vi "PR_Update_screw_eve_result.vi"(8 "result":string, 9 "data":T1, 10 "barcode":string="984132195", 11 "DBlink":string="Driver={ODBC Driver 17 for SQL Server};Server=localhost\\SQLEXPRESS;Database=ZDX201;UID=labview;PWD=Dsa@54137926") -> (0 "error out":errorcluster)   [LabVIEW 2019]
uses:
  <vilib>/addons/database/Connection.llb/DB Tools Open Connec (String).vi
  <vilib>/addons/database/NI_Database_API.lvlib
panel:
  out "concatenated string":string="WHERE [barcode]='984132195' and [pos]='B'"
  in  "error in (no error)":errorcluster
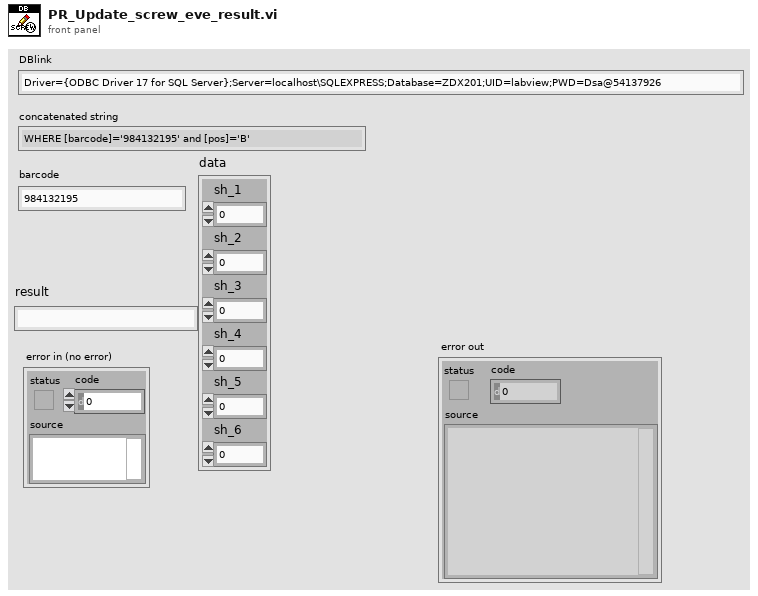
[diagram p1: front panel]
types:
  T1 = cluster{"sh_1":dbl, "sh_2":dbl, "sh_3":dbl, "sh_4":dbl, "sh_5":dbl, "sh_6":dbl}
  T2 = cluster{"done_time3":timestamp, "update_time":timestamp, "result":string, "sh_1":dbl, "sh_2":dbl, "sh_3":dbl, "sh_4":dbl, "sh_5":dbl, "sh_6":dbl}
  T3 = typedef "NI_Database_API.lvlib/Conn ObjectReference.ctl" = refnum<k1>
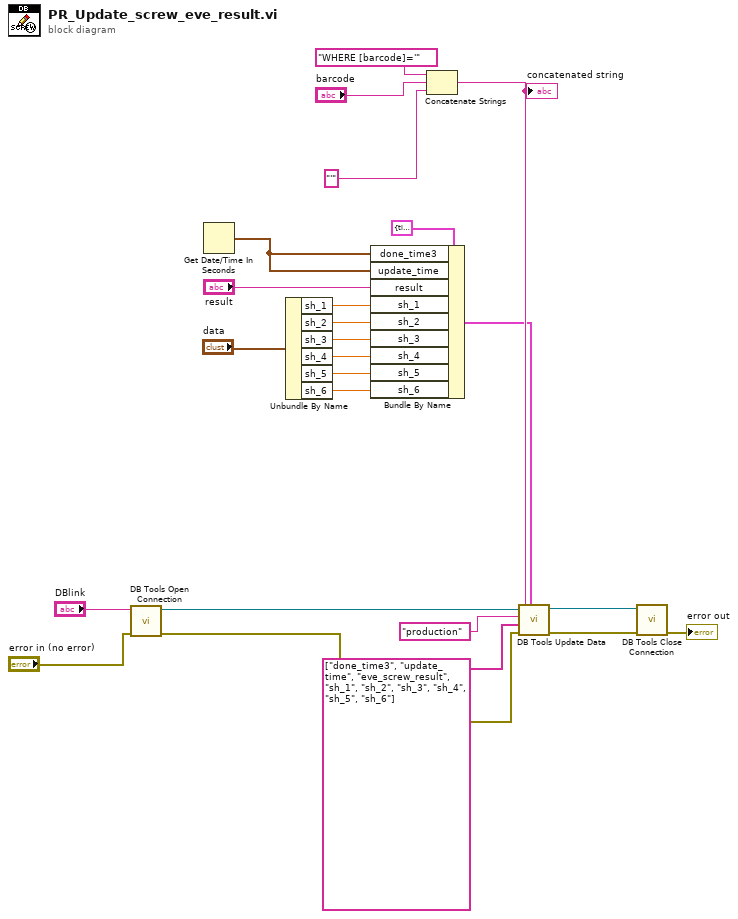
[diagram p0: block diagram]
diagram:
  n1 = call-poly <vilib>:"DB Tools Open Connection.vi"("error in (no error)"="error in (no error)", "connection information"="DBlink") -> ("error out"=w22:errorcluster, "connection reference"=w20:T3)  [unwired: 6 in]
  n2 = Get Date/Time In Seconds() -> (seconds since 1Jan1904=w11:timestamp)
  n3 = Unbundle By Name("data") -> ("sh_1"=w6:dbl, "sh_2"=w5:dbl, "sh_3"=w4:dbl, "sh_4"=w3:dbl, "sh_5"=w2:dbl, "sh_6"=w1:dbl)
  n4 = Bundle By Name(cluster=T2 {"done_time3"=timestamp(0 s since 1904-01-01), "update_time"=timestamp(0 s since 1904-01-01), "result"="", "sh_1"=0.0, "sh_2"=0.0, "sh_3"=0.0, "sh_4"=0.0, "sh_5"=0.0, "sh_6"=0.0}, "done_time3"=w11, "update_time"=w11, "result"="result", "sh_1"=w6, "sh_2"=w5, "sh_3"=w4, "sh_4"=w3, "sh_5"=w2, "sh_6"=w1) -> (w10:T2)
  n5 = Concatenate Strings("WHERE [barcode]='", "barcode", "'" ("string")) -> (w14:string)
  "concatenated string" <- w14
  n6 = call <vilib>:"DB Tools Update Data.vi"("condition"=w14, "data"=w10, "error in (no error)"=w22, "columns"=string[] ["done_time3", "update_time", "eve_screw_result", "sh_1", "sh_2", "sh_3", "sh_4", "sh_5", "sh_6"], "table"="production", "connection reference"=w20) -> ("error out"=w23:errorcluster, "connection reference out"=w21:T3)  [unwired: 4 in]
  n7 = call <vilib>:"DB Tools Close Connection.vi"("error in (no error)"=w23, "connection reference"=w21) -> ("error out"=→"error out":errorcluster)  [unwired: 5 in]
